vi "Handle1.vi"(8 "error in (no error)":errorcluster, 11 "Acquisition in":refnum<class "Acquisition.lvclass">) -> (0 "error out":errorcluster, 3 "Acquisition out":refnum<class "Acquisition.lvclass">)   [LabVIEW 2018, in "Acquisition.lvclass"]
uses:
  Acquisition.lvclass
  Acquisition.lvclass/Acquisition.ctl
  Comm/Stream/Stream.lvclass
  Channel/Channel.lvclass
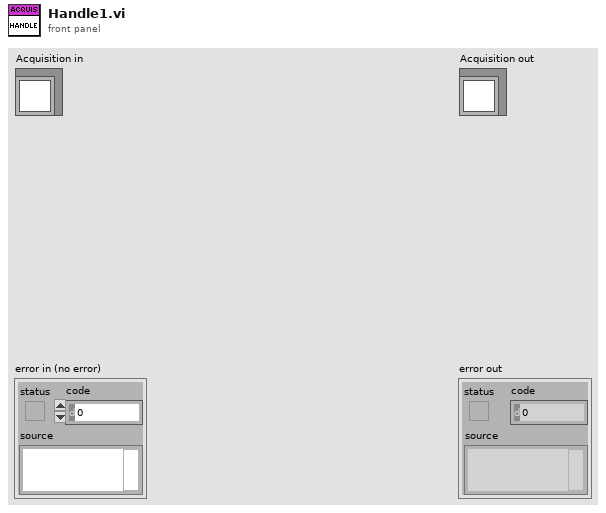
[diagram p1: front panel]
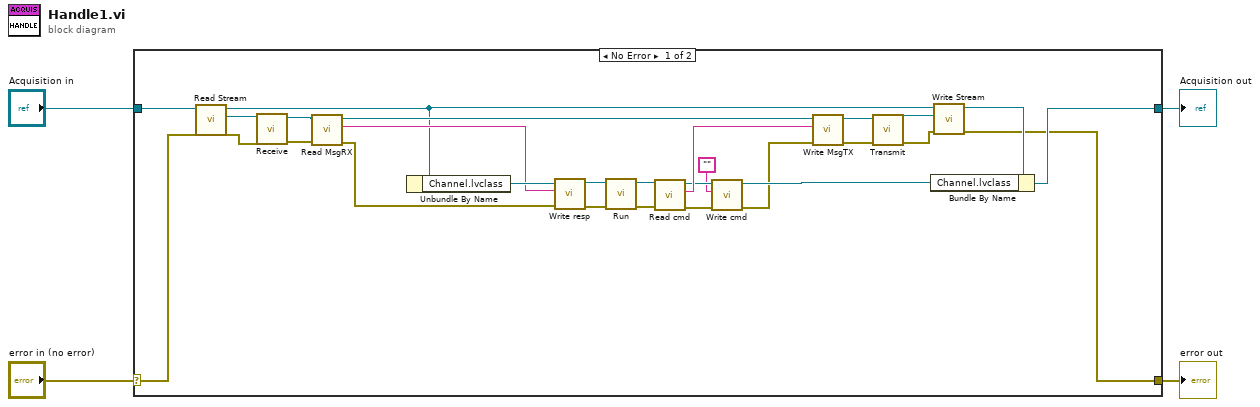
[diagram p0: block diagram]
diagram:
  n1 = case shown="No Error" "error in (no error)" {
    selector: "error in (no error)" -> [w29 w34]
    tunnel: [w12 w34] -> w3
    tunnel: [w26 w33] -> w1
    tunnel: "Acquisition in" -> [w32 w33]
    frame No Error {
      n2 = call-dynamic "Read Stream.vi"("error in (no error)"=w29, "Server in"=w32) -> ("error out"=w30:errorcluster, "Stream.lvclass"=w31:refnum<class "Stream.lvclass">, "Server out"=w16:refnum<class "Acquisition.lvclass">)  [unwired: 7 in]
      n3 = call-dynamic "Receive.vi"("error in (no error)"=w30, "Stream in"=w31) -> ("error out"=w25:errorcluster, "Stream out"=w24:refnum<class "Stream.lvclass">)  [unwired: 8 in]
      n4 = call-dynamic "Read MsgRX.vi"("error in (no error)"=w25, "Comm in"=w24) -> ("error out"=w22:errorcluster, "MsgRX"=w23:string, "Comm out"=w21:refnum<class "Stream.lvclass">)  [unwired: 7 in]
      n5 = Unbundle By Name(w16) -> ("Channel.lvclass"=w28:refnum<class "Channel.lvclass">)
      n6 = call-dynamic "Write resp.vi"("error in (no error)"=w22, "resp"=w23, "Device in"=w28) -> ("error out"=w11:errorcluster, "Device out"=w10:refnum<class "Channel.lvclass">)  [unwired: 7 in]
      n7 = call-dynamic "Run.vi"("error in (no error)"=w11, "Channel in"=w10) -> ("error out"=w8:errorcluster, "Channel out"=w9:refnum<class "Channel.lvclass">)  [unwired: 8 in]
      n8 = call-dynamic "Read cmd.vi"("error in (no error)"=w8, "Device in"=w9) -> ("error out"=w6:errorcluster, "cmd"=w20:string, "Device out"=w7:refnum<class "Channel.lvclass">)  [unwired: 7 in]
      n9 = call-dynamic "Write cmd.vi"("error in (no error)"=w6, "cmd"="", "Device in"=w7) -> ("error out"=w19:errorcluster, "Device out"=w27:refnum<class "Channel.lvclass">)  [unwired: 7 in]
      n10 = call-dynamic "Write MsgTX.vi"("error in (no error)"=w19, "MsgTX"=w20, "Comm in"=w21) -> ("error out"=w17:errorcluster, "Comm out"=w18:refnum<class "Stream.lvclass">)  [unwired: 7 in]
      n11 = call-dynamic "Transmit.vi"("error in (no error)"=w17, "Stream in"=w18) -> ("error out"=w13:errorcluster, "Stream out"=w15:refnum<class "Stream.lvclass">)  [unwired: 8 in]
      n12 = call-dynamic "Write Stream.vi"("error in (no error)"=w13, "Stream.lvclass"=w15, "Server in"=w16) -> ("error out"=w12:errorcluster, "Server out"=w14:refnum<class "Acquisition.lvclass">)  [unwired: 7 in]
      n13 = Bundle By Name(cluster=w14, "Channel.lvclass"=w27) -> (w26:refnum<class "Acquisition.lvclass">)
    }
    frame Error {
    }
  }
  "error out" <- w3
  "Acquisition out" <- w1
